vi "tm482_electroncoefficient_wVision.vi"() -> ()   [LabVIEW 2023, in "HamamatsuCam.lvlib" / "HamamatsuCam.lvclass"]
uses:
  HamamatsuCam/HamamatsuCam/HamamatsuCam.lvclass
panel:
  out "Photons":sgl format="%.2f"
  out "Display":T1(plugin-control)
  out "Offset":sgl
  out "Coefficient":sgl
  out "Frames Per Second":dbl
  in  "Quit":bool
  out "Error Out":errorcluster
  # "This is an example on how to get\nthe electron count value where \nthe mouse cursor is on the image."
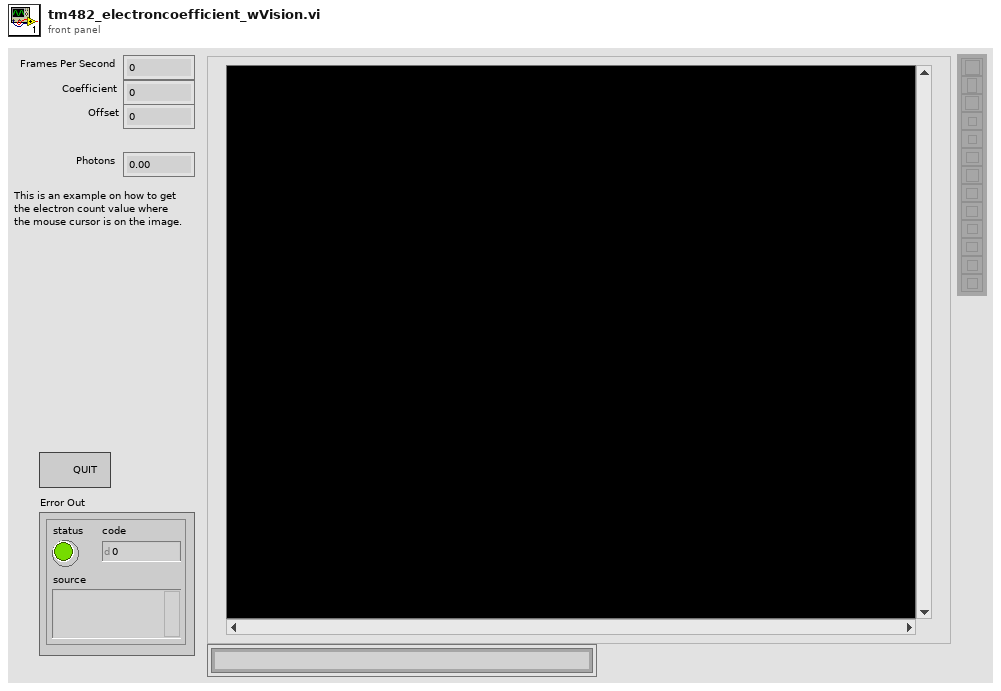
[diagram p1: front panel]
types:
  T1 = typedef "IMAQ Image.ctl" = refnum<image>
  T2 = typedef "Image Type" = u32
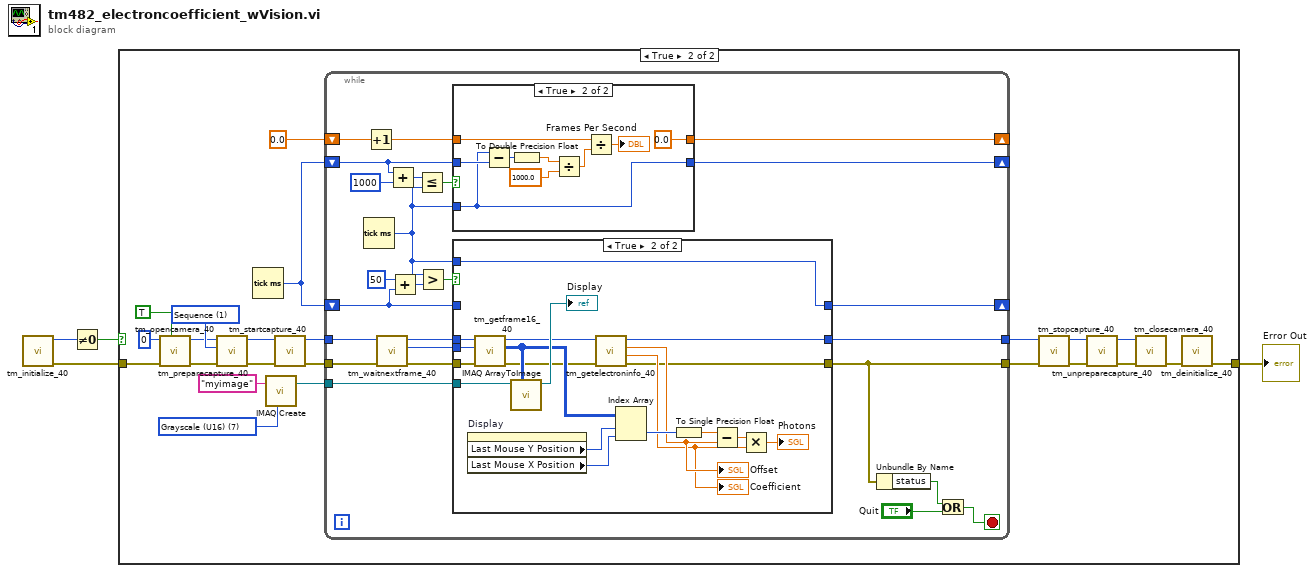
[diagram p0: block diagram]
diagram:
  n1 = call "tm_initialize_40.vi"() -> ("error out"=w1:errorcluster, "Number Of Cameras"=w2:u32)  [unwired: 8 in, 2 out]
  n2 = Not Equal To 0?(x=w2) -> (x != 0?=w4:bool)
  n3 = case shown="True" w4 {
    tunnel: w1 -> [w5 w28]
    tunnel: [w5 w25] -> w3
    frame False {
    }
    frame True {
      w9 = T2 7 items=["Grayscale (U8)", "Grayscale (I16)", "Grayscale (SGL)", "Complex (CSG)", "RGB (U32)", "HSL (U32)", "RGB (U64)", "Grayscale (U16)"] ("Image Type")
      w16 = 1 items=["Snap", "Sequence"] ("Capture mode")
      n4 = call "tm_opencamera_40.vi"("Force Open"=TRUE, "error in (no error)"=w28, "Camera Index"=u32 0) -> ("error out"=w10:errorcluster, "Handle out"=w11:u32)  [unwired: 6 in, 1 out]
      n5 = call "tm_preparecapture_40.vi"("error in (no error)"=w10, "Capture mode"=w16, "Handle in"=w11) -> ("error out"=w14:errorcluster, "Handle out"=w15:u32)  [unwired: 5 in, 2 out]
      n6 = Tick Count (ms)() -> (millisecond timer value=w12:u32)
      n7 = call "IMAQ Create"("Image Name"="myimage", "Image Type"=w9) -> ("New Image"=w8:T1)  [unwired: 3 in, 1 out]
      n8 = call "tm_startcapture_40.vi"("error in (no error)"=w14, "Handle in"=w15) -> ("error out"=w17:errorcluster, "Handle out"=w18:u32)  [unwired: 8 in]
      n9 = while {
        tunnel: [w32] -> w21
        tunnel: [w33] -> w22
        tunnel: w18 -> [w50]
        tunnel: w17 -> [w51]
        shift-right: [w48] -> _
        shift-left: w12 -> [w45]
        shift-right: [w49] -> _
        shift-left: 0.0 -> [w42]
        shift-right: [w31] -> _
        shift-left: w12 -> [w34]
        tunnel: w8 -> [w30]
        stop <- w29 stop-if-true
        n10 = Tick Count (ms)() -> (millisecond timer value=w35:u32)
        n11 = Increment(x=w42) -> (x+1=w43:dbl)
        n12 = call "tm_waitnextframe_40.vi"("error in (no error)"=w51, "Handle in"=w50) -> ("error out"=w40:errorcluster, "Frame Index"=w39:i32, "Handle out"=w41:u32)  [unwired: 6 in, 1 out]
        n13 = Add(x=w45, y=u32 1000) -> (x+y=w47:u32)
        n14 = Add(x=u32 50, y=w34) -> (x+y=w37:u32)
        n15 = Less Or Equal?(x=w47, y=w35) -> (x <= y?=w44:bool)
        n16 = Greater?(x=w35, y=w37) -> (0:w36:bool)
        n17 = case shown="True" w44 {
          tunnel: w45 -> [w77 w80]
          tunnel: [w77 w78] -> w48
          tunnel: w43 -> [w76 w84]
          tunnel: w35 -> [_ w78]
          tunnel: [w76 0.0] -> w49
          frame False {
          }
          frame True {
            n18 = Subtract(x=w78, y=w80) -> (x-y=w79:u32)
            n19 = To Double Precision Float(number=w79) -> (double precision float=w86:dbl)
            n20 = Divide(x=w86, y=1000.0) -> (x/y=w83:dbl)
            n21 = Divide(x=w84, y=w83) -> (x/y=→"Frames Per Second":dbl)
          }
        }
        n22 = case shown="True" w36 {
          tunnel: w41 -> [w56 w62]
          tunnel: w40 -> [w55 w61]
          tunnel: w39 -> [_ w66]
          tunnel: w34 -> [w54 _]
          tunnel: w35 -> [_ w75]
          tunnel: [w56 w57] -> w32
          tunnel: [w55 w58] -> w33
          tunnel: [w54 w75] -> w31
          tunnel: w30 -> [_ w74]
          frame False {
          }
          frame True {
            n23 = property on="Display" class="ImageControl"() -> ("Last Mouse Y Position"=w67:i32, "Last Mouse X Position"=w63:i32)  [unwired: 2 in, 2 out]
            n24 = call "tm_getframe16_40.vi"("error in (no error)"=w61, "Frame Index"=w66, "Handle in"=w62) -> ("error out"=w59:errorcluster, "Data"=w72:u16[][], "Handle out"=w60:u32)  [unwired: 5 in, 1 out]
            n25 = call "IMAQ ArrayToImage"("Image Pixels (U16)"=w72, "Image"=w74) -> ("Image Out"=→"Display":T1)  [unwired: 8 in, 1 out]
            n26 = call "tm_getelectroninfo_40.vi"("error in (no error)"=w59, "Handle in"=w60) -> ("error out"=w58:errorcluster, "Coefficient"=w64:sgl, "Offset"=w65:sgl, "Handle out"=w57:u32)  [unwired: 6 in]
            "Coefficient" <- w64
            "Offset" <- w65
            n27 = Index Array(array=w72, index (row)=w67, index (col)=w63) -> (element=w70:u16)
            n28 = To Single Precision Float(number=w70) -> (single precision float=w69:sgl)
            n29 = Subtract(x=w69, y=w65) -> (x-y=w71:sgl)
            n30 = Multiply(x=w71, y=w64) -> (x*y=→"Photons":sgl)
          }
        }
        n31 = Unbundle By Name(w33) -> ("status"=w53:bool)
        n32 = Or(x=w53, y="Quit") -> (x .or. y?=w29:bool)
      }
      n33 = call "tm_stopcapture_40.vi"("error in (no error)"=w22, "Handle in"=w21) -> ("error out"=w19:errorcluster, "Handle out"=w20:u32)  [unwired: 8 in]
      n34 = call "tm_unpreparecapture_40.vi"("error in (no error)"=w19, "Handle in"=w20) -> ("error out"=w24:errorcluster, "Handle out"=w23:u32)  [unwired: 8 in]
      n35 = call "tm_closecamera_40.vi"("error in (no error)"=w24, "Handle in"=w23) -> ("error out"=w26:errorcluster)  [unwired: 9 in]
      n36 = call "tm_deinitialize_40.vi"("error in (no error)"=w26) -> ("error out"=w25:errorcluster)  [unwired: 10 in]
    }
  }
  "Error Out" <- w3
